vi "Get Pin Map Service Address.vi"(8 "error in (no error)":errorcluster) -> (0 "error out":errorcluster, 3 "address":string)   [LabVIEW 2020]
uses:
  Discovery Client_lv/MeasurementLink Discovery Client/RPC Messages/ni_measurementlink_discovery_v1_ResolveServiceRequest.ctl
  Discovery Client_lv/MeasurementLink Discovery Client/MeasurementLink Discovery Client.lvlib
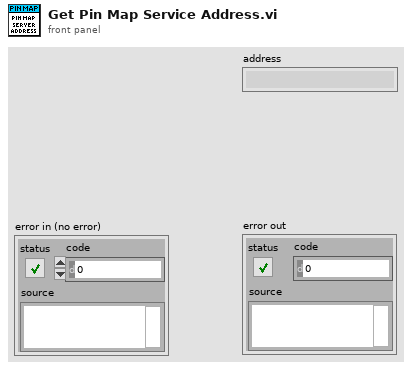
[diagram p1: front panel]
types:
  T1 = typedef "MeasurementLink Discovery Client.lvlib/ni_measurementlink_discovery_v1_ResolveServiceRequest.ctl" = cluster{"provided_interface":string, "service_class":string}
  T2 = typedef "MeasurementLink Discovery Client.lvlib/ni_measurementlink_discovery_v1_ServiceLocation.ctl" = cluster{"location":string, "insecure_port":string, "ssl_authenticated_port":string}
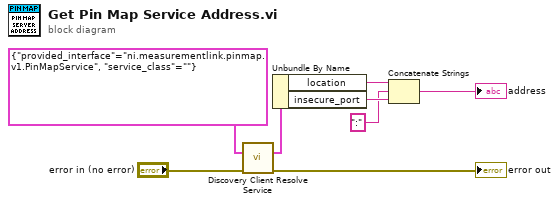
[diagram p0: block diagram]
diagram:
  n1 = call "Discovery Client Resolve Service.vi"("Request Data"=T1 {"provided_interface"="ni.measurementlink.pinmap.v1.PinMapService", "service_class"=""}, "error in (no error)"="error in (no error)") -> ("Response Data"=w5:T2, "error out"=→"error out":errorcluster)  [unwired: 12 in]
  n2 = Unbundle By Name(w5) -> ("location"=w4:string, "insecure_port"=w3:string)
  n3 = Concatenate Strings(w4, ":" ("string"), w3) -> (→"address":string)
